vi "mqttCmdBuildPayload.vi"(0 "mqttConnect in":refnum<class "mqttCmdConnect.lvclass">, 11 "error in (no error)":errorcluster) -> (4 "mqttConnect out":refnum<class "mqttCmdConnect.lvclass">, 8 "payload":u8[](array[numeric]) format="%x", 15 "error out":errorcluster)   [LabVIEW 2018, in "mqttCmdConnect.lvclass"]
uses:
  mqttCmdConnect.lvclass
  mqttCmdConnect.lvclass/mqttCmdConnect.ctl
  mqtt.lvclass
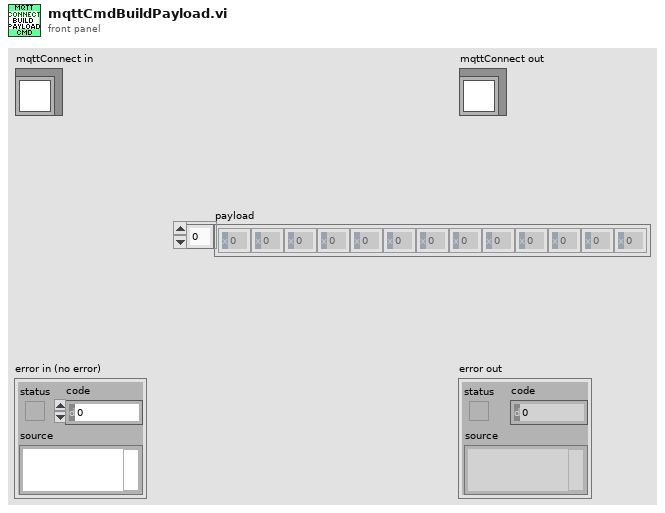
[diagram p1: front panel]
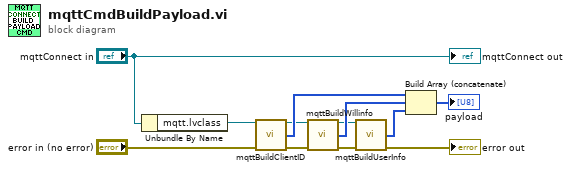
[diagram p0: block diagram]
diagram:
  n1 = Unbundle By Name("mqttConnect in") -> ("mqtt.lvclass"=w1:refnum<class "mqtt.lvclass">)
  n2 = call "mqttBuildClientID.vi"("mqtt in"=w1, "error in (no error)"="error in (no error)") -> ("mqtt out"=w11:refnum<class "mqtt.lvclass">, "clientID out"=w12:u8[], "error out"=w10:errorcluster)  [unwired: 11 in]
  n3 = call "mqttBuildWillinfo.vi"("mqtt in"=w11, "error in (no error)"=w10) -> ("mqtt out"=w7:refnum<class "mqtt.lvclass">, "willMessage out"=w9:u8[], "error out"=w8:errorcluster)  [unwired: 11 in]
  n4 = call "mqttBuildUserInfo.vi"("mqtt in"=w7, "error in (no error)"=w8) -> ("userInfo out"=w6:u8[], "error out"=→"error out":errorcluster)  [unwired: 11 in, 1 out]
  n5 = Build Array (concatenate)(w12, w9, w6) -> (→"payload":u8[])
  "mqttConnect out" <- "mqttConnect in"
